vi "benchmarks_smallBinaryMD5.vi"() -> ()   [LabVIEW 2013]
uses:
  MD5/MD5.lvclass
  <vilib>/Analysis/baseanly.llb/Mean (DBL).vi
  MD5/MD5.lvlib
  <vilib>/Analysis/NI_AALBase.lvlib
panel:
  out "% gain":dbl
  out "LVOS":dbl
  out "NI":dbl
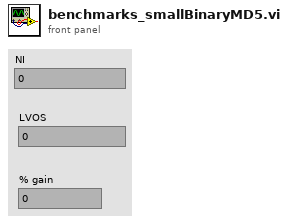
[diagram p1: front panel]
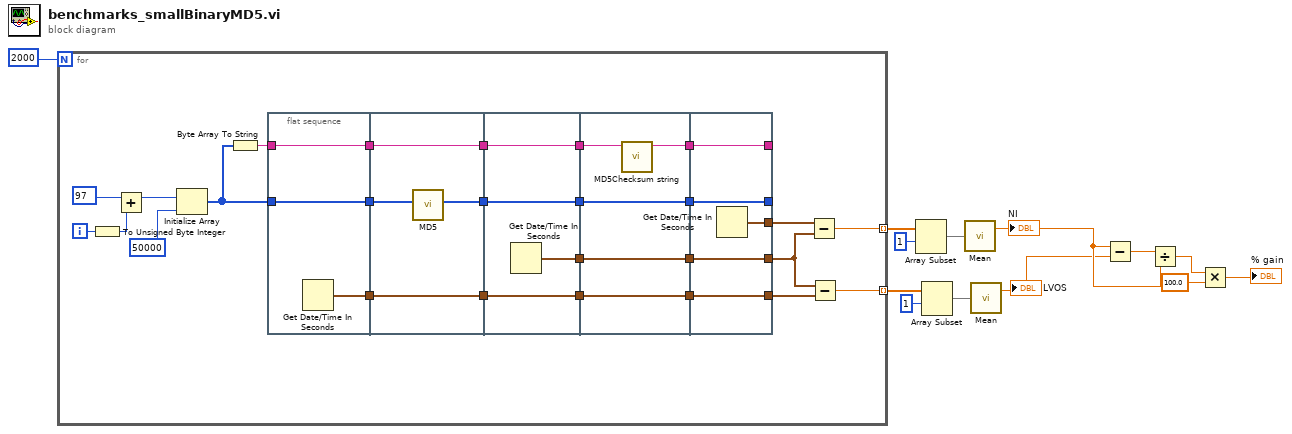
[diagram p0: block diagram]
diagram:
  n1 = for {
    N: 2000 -> [_]
    tunnel: [w25] -> w12 mode=indexing
    tunnel: [w24] -> w7 mode=indexing
    i -> [w14]
    n2 = To Unsigned Byte Integer(number=w14) -> (unsigned 8bit integer=w15:u8)
    n3 = Add(x=u8 97 ("Numeric"), y=w15) -> (x+y=w16:u8)
    n4 = Initialize Array(w16, 50000 ("dimension size")) -> (w21:u8[])
    n5 = Byte Array To String(unsigned byte array=w21) -> (string=w22:string)
    n6 = flat-sequence {
      tunnel: [w42] -> w39
      tunnel: w21 -> [w41]
      tunnel: [w41] -> w38
      tunnel: w22 -> [w40]
      tunnel: [w40] -> w37
      tunnel: w39 -> [w46]
      tunnel: [w46] -> w36
      tunnel: [w44] -> w35
      tunnel: w38 -> [w45]
      tunnel: w37 -> [w43]
      tunnel: [w43] -> w34
      tunnel: [w50] -> w33
      tunnel: [w49] -> w32
      tunnel: w36 -> [w49]
      tunnel: [w48] -> w31
      tunnel: w35 -> [w48]
      tunnel: w34 -> [w47]
      tunnel: [w47] -> w30
      tunnel: [w55] -> w29
      tunnel: w33 -> [w55]
      tunnel: [w54] -> w28
      tunnel: w32 -> [w54]
      tunnel: [w52] -> w27
      tunnel: [w53] -> w26
      tunnel: w31 -> [w53]
      tunnel: w30 -> [w51]
      tunnel: [w60] -> w19
      tunnel: w29 -> [w60]
      tunnel: [w59] -> w18
      tunnel: w28 -> [w59]
      tunnel: [w58] -> w20
      tunnel: [w57] -> _
      tunnel: w27 -> [w57]
      tunnel: [w56] -> _
      tunnel: w26 -> [w56]
      frame #0 {
        n7 = Get Date/Time In Seconds() -> (seconds since 1Jan1904=w42:timestamp)
      }
      frame #1 {
        n8 = call "MD5.vi"("data"=w45) -> ("MD5 hash"=w44:u8[])  [unwired: 10 in]
      }
      frame #2 {
        n9 = Get Date/Time In Seconds() -> (seconds since 1Jan1904=w50:timestamp)
      }
      frame #3 {
        n10 = call <vilib>:"MD5Checksum string.vi"("Message String"=w51) -> ("MD5 message-digest"=w52:string)  [unwired: 10 in]
      }
      frame #4 {
        n11 = Get Date/Time In Seconds() -> (seconds since 1Jan1904=w58:timestamp)
      }
    }
    n12 = Subtract(x=w20, y=w19) -> (x-y=w25:dbl)
    n13 = Subtract(x=w19, y=w18) -> (x-y=w24:dbl)
  }
  n14 = Array Subset(array=w12, index=1) -> (w10:dbl[])  [unwired: 1 in]
  n15 = Array Subset(array=w7, index=1) -> (w9:dbl[])  [unwired: 1 in]
  n16 = call-poly <vilib>:"Mean.vi"("X"=w10) -> ("mean"=w2:dbl)  [unwired: 1 out]
  "NI" <- w2
  n17 = call-poly <vilib>:"Mean.vi"("X"=w9) -> ("mean"=w1:dbl)  [unwired: 1 out]
  "LVOS" <- w1
  n18 = Subtract(x=w2, y=w1) -> (x-y=w6:dbl)
  n19 = Divide(x=w6, y=w2) -> (x/y=w4:dbl)
  n20 = Multiply(x=w4, y=100.0) -> (x*y=→"% gain":dbl)
